vi "checkPC.vi"() -> (0 "error out":errorcluster, 2 "All on?":bool, 3 "Computers not on":string[](array[string]))   [LabVIEW 2020]
uses:
  Shared/MySQL/Preset Query Enum.ctl
  <userlib>/_OpenG.lib/array/array.llb/Remove Duplicates from 1D Array (String)__ogtk.vi
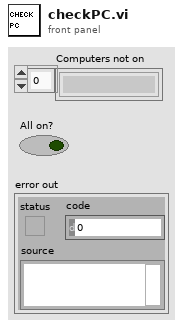
[diagram p1: front panel]
types:
  T1 = typedef "Preset Query Enum.ctl" = enum16{"Get Locations", "Get all IPs and MACs", "Get classes", "Get expt variables to set at scanstart for particular device", "Get expt devices and variables with start values", "Get expt devices and variables (with data to get)", "Get expt devices with data to get", "Get Expt devices and GUIs", "Get all devices basic properties", "Get Virtual Devices Core Info", "Get Expt names", "Get experiment basic properties", "Get experiment alarm variables", "Get MC Ports", "Get device network comm port", "Get devicetype lvclass path", "Get basic device properties", "Get Init Order", "Get all setable variables of a device", "Get device variable aliases", "Get force values of all settable variables", "Get all variables of a devicetype", "Get all variables of a device", "Get plotter details", "Get Saved Scans", "Get Scan Info", "GetGeneralGUIs", "Get expt for plotter", "Get plotter IDs from expt", "Get all devices", "Get all Virtual Devices", "Get all aliases", "Get variable and device info for Virtual Device", "GetItemLocatorIP", "Get IPs for GUIs", "Get DeviceType from Device", "GetLocalPortRange", "GetDevicePresetVariables", "Get Device Configuration", "GetAllPresetNames", "GetAllConfigurationNames", "GetPresetDeviceNames", "GetDeviceAliases", "GetDevicesOfClass"}
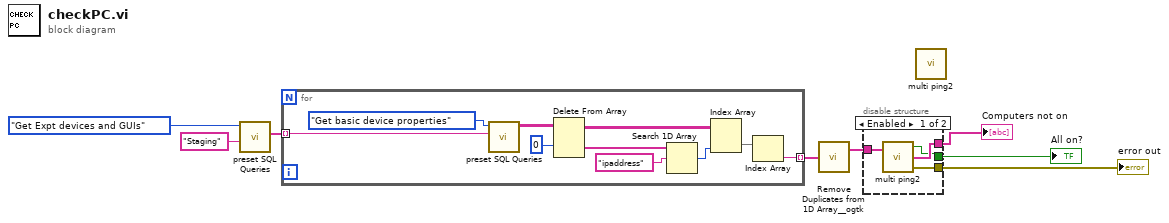
[diagram p0: block diagram]
diagram:
  n1 = call "preset SQL Queries.vi"("Expt name / MCIP/ Variable/Preset Name"="Staging" ("Expt name / MCIP/ Variable Name"), "Preset Query"=Preset_Query_Enum."Get Expt devices and GUIs") -> ("1st column 1st data"=w5:string[])  [unwired: 7 in, 2 out]
  n2 = for {
    tunnel: w5 -> [w17] mode=indexing
    tunnel: [w9] -> w4 mode=indexing
    n3 = call "preset SQL Queries.vi"("Device/Devicetype name\n/Plotter.id/ScanName#"=w17, "Preset Query"=Preset_Query_Enum."Get basic device properties") -> ("data"=w13:string[][])  [unwired: 7 in, 2 out]
    n4 = Delete From Array(array=w13, index (row)=0) -> (deleted portion=w15:string[], array with subset deleted=w11:string[][])  [unwired: 2 in]
    n5 = Search 1D Array(1D array=w15, element="ipaddress") -> (index of element=w12:i32)  [unwired: 1 in]
    n6 = Index Array(array=w11, index (col)=w12) -> (element=w10:string[])  [unwired: 1 in]
    n7 = Index Array(array=w10) -> (element=w9:string)  [unwired: 1 in]
  }
  n8 = call-poly <userlib>:"Remove Duplicates from 1D Array__ogtk.vi"("Input Array"=w4) -> ("Output Array"=w3:string[])  [unwired: 1 out]
  n9 = disable-structure shown="Enabled" {
    disable-tunnel: [w22 _] -> w1
    disable-tunnel: [w21 _] -> w2
    disable-tunnel: w3 -> [w20 _]
    disable-tunnel: [w19 _] -> w8
    frame Enabled {
      n10 = call "multi ping2.vi"("IP Addresses"=w20) -> ("All on?"=w21:bool, "Computers not on"=w22:string[], "error out"=w19:errorcluster)  [unwired: 1 in]
    }
    frame Disabled {
    }
  }
  "error out" <- w8
  "All on?" <- w2
  "Computers not on" <- w1
  n11 = call "multi ping2.vi"() -> ()  [unwired: 2 in, 3 out]
